vi "Application Paths.vi"(0 "gScript Interpreter in":refnum<class "gScript Interpreter.lvclass">, 5 "error in (no error)":errorcluster) -> (14 "gScript Interpreter out":refnum<class "gScript Interpreter.lvclass">, 15 "Project Path":path, 16 "Config Path":path, 17 "Scripts Path":path, 18 "Logs Path":path, 19 "error out":errorcluster)   [LabVIEW 2023, in "gScript Interpreter.lvclass"]
uses:
  gScript Interpreter.lvclass
  gScript Interpreter.lvclass/gScript Interpreter.ctl
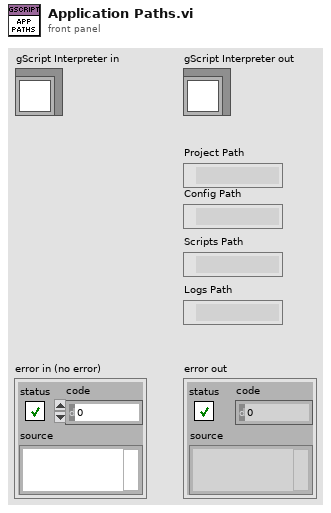
[diagram p1: front panel]
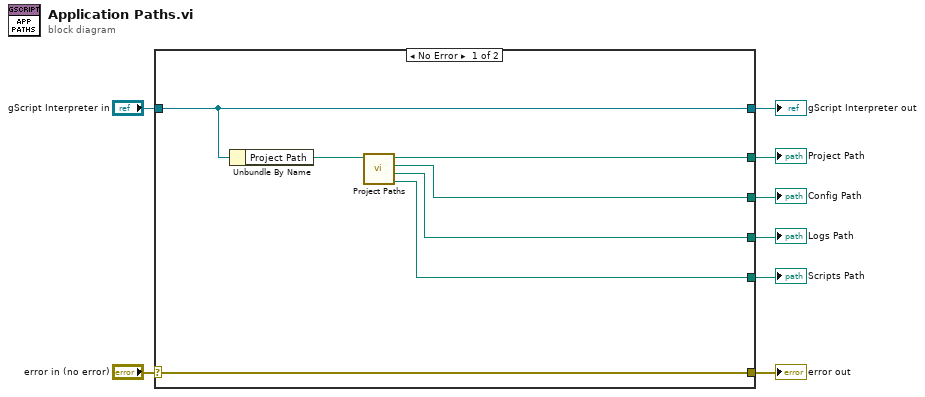
[diagram p0: block diagram]
diagram:
  n1 = case shown="No Error" "error in (no error)" {
    selector: "error in (no error)" -> [w15 w17]
    tunnel: [w15 w17] -> w7
    tunnel: [w14 w16] -> w5
    tunnel: "gScript Interpreter in" -> [w14 w16]
    tunnel: [w12 _] -> w4
    tunnel: [w10 _] -> w3
    tunnel: [w9 _] -> w2
    tunnel: [w11 _] -> w1
    frame No Error {
      n2 = Unbundle By Name(w14) -> ("Project Path"=w13:path)
      n3 = call "Project Paths.vi"("Project Path in"=w13) -> ("Scripts Path"=w9:path, "Logs Path"=w10:path, "Config Path"=w11:path, "Project Path"=w12:path)  [unwired: 6 in, 1 out]
    }
    frame Error {
    }
  }
  "error out" <- w7
  "gScript Interpreter out" <- w5
  "Config Path" <- w1
  "Scripts Path" <- w2
  "Logs Path" <- w3
  "Project Path" <- w4
